vi "Calculate Button Dialog Parameters.vi"(1 "Max Message Indicator Width":dbl, 5 "bottom":i16, 7 "top":i16, 9 "right":i16) -> (4 "Indicator left position":dbl, 6 "Calculated indicator height":dbl, 8 "Indicator height scaled large":dbl, 10 "Actual indicator height":dbl, 15 "Indicator height scaled small":dbl)   [LabVIEW 2010]
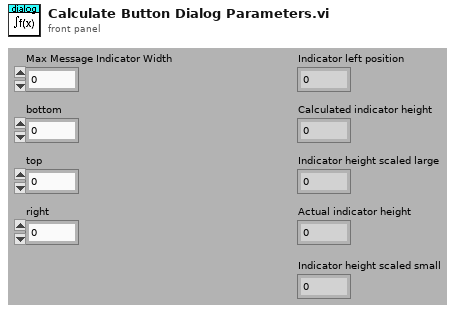
[diagram p1: front panel]
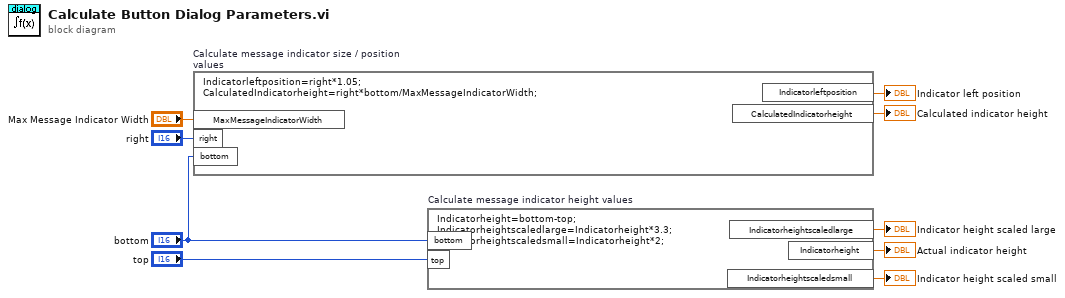
[diagram p0: block diagram]
diagram:
  n1 = formula code="Indicatorleftposition=right*1.05;\nCalculatedIndicatorheight=right*bottom/MaxMessageIndicatorWidth;" "Calculate message indicator size / position values"("right"="right", "bottom"="bottom", "MaxMessageIndicatorWidth"="Max Message Indicator Width") -> ("CalculatedIndicatorheight"=→"Calculated indicator height":dbl, "Indicatorleftposition"=→"Indicator left position":dbl)
  n2 = formula code="Indicatorheight=bottom-top;\nIndicatorheightscaledlarge=Indicatorheight*3.3;\nIndicatorheightscaledsmall=Indicatorheight*2;" "Calculate message indicator height values"("bottom"="bottom", "top"="top") -> ("Indicatorheight"=→"Actual indicator height":dbl, "Indicatorheightscaledlarge"=→"Indicator height scaled large":dbl, "Indicatorheightscaledsmall"=→"Indicator height scaled small":dbl)
